vi "Save Material Theme.vi"(8 "error in":errorcluster, 10 "Theme":refnum<class "Material Theme.lvclass">, 11 "file path":path) -> (0 "error out":errorcluster, 1 "text":string)   [LabVIEW 2021, in "TSC Material Theme.lvlib" / "Material Theme.lvclass"]
doc: "Save a material theme from to disk in a JSON file format.\n\n<b>Code Developed By:</b> +\nTechnology Service Corporation +\nwww.tsc.com/atcs\n\nDeveloper:\nDaniel Coons"
uses:
  Material Theme.lvclass
  Material Theme.lvclass/Material Theme.ctl
  <vilib>/JDP Science/JSONtext/LVClass Serializer/JSONtext LVClass Serializer.lvclass
  TSC Material Theme.lvlib
  Material-Scheme/Material-Scheme.lvclass
  Material-Palette/Material-Palette.lvclass
  <vilib>/JDP Science/JSONtext/JSONtext.lvlib
  6cf305a8-b973-47b4-be4a-a40db0a30ff0.vi
panel:
  # "FOR DEBUG"
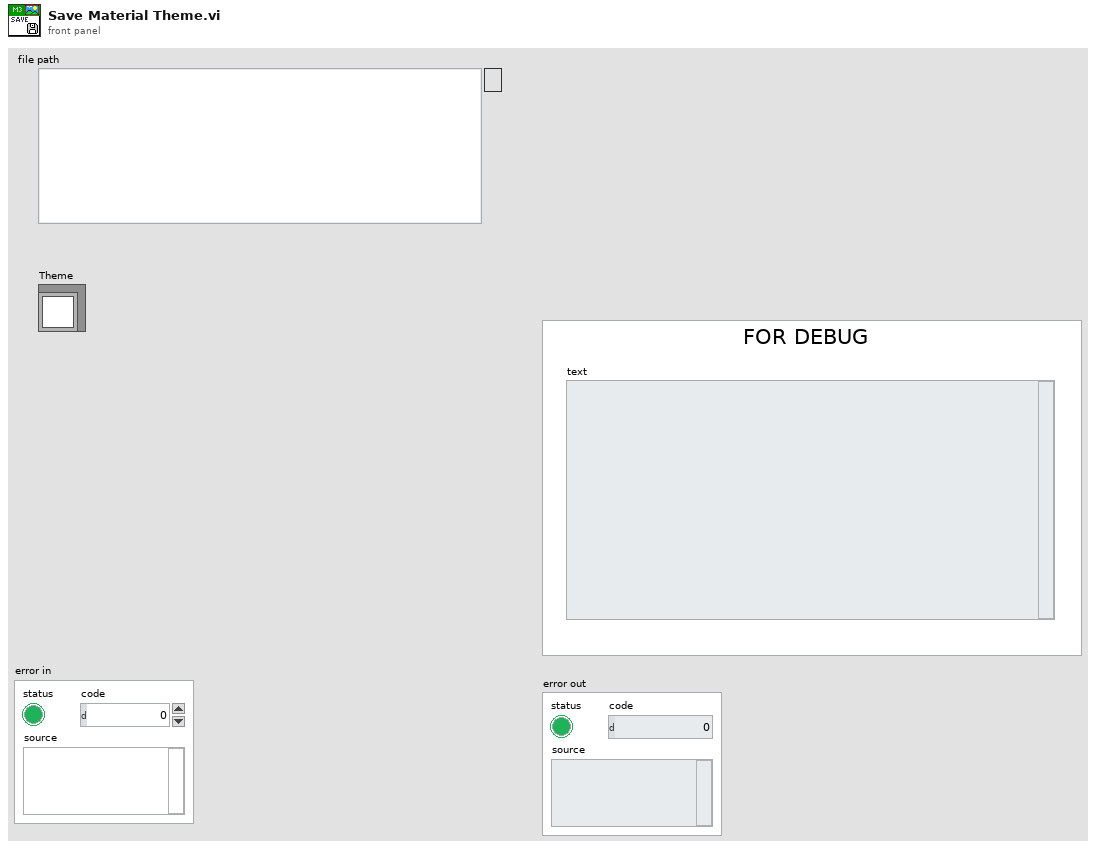
[diagram p1: front panel]
types:
  T1 = enum16{"open", "replace", "create", "open or create", "replace or create", "replace or create with confirmation"}
  T2 = cluster{"primary":u32, "secondary":u32, "tertiary":u32, "error":u32}
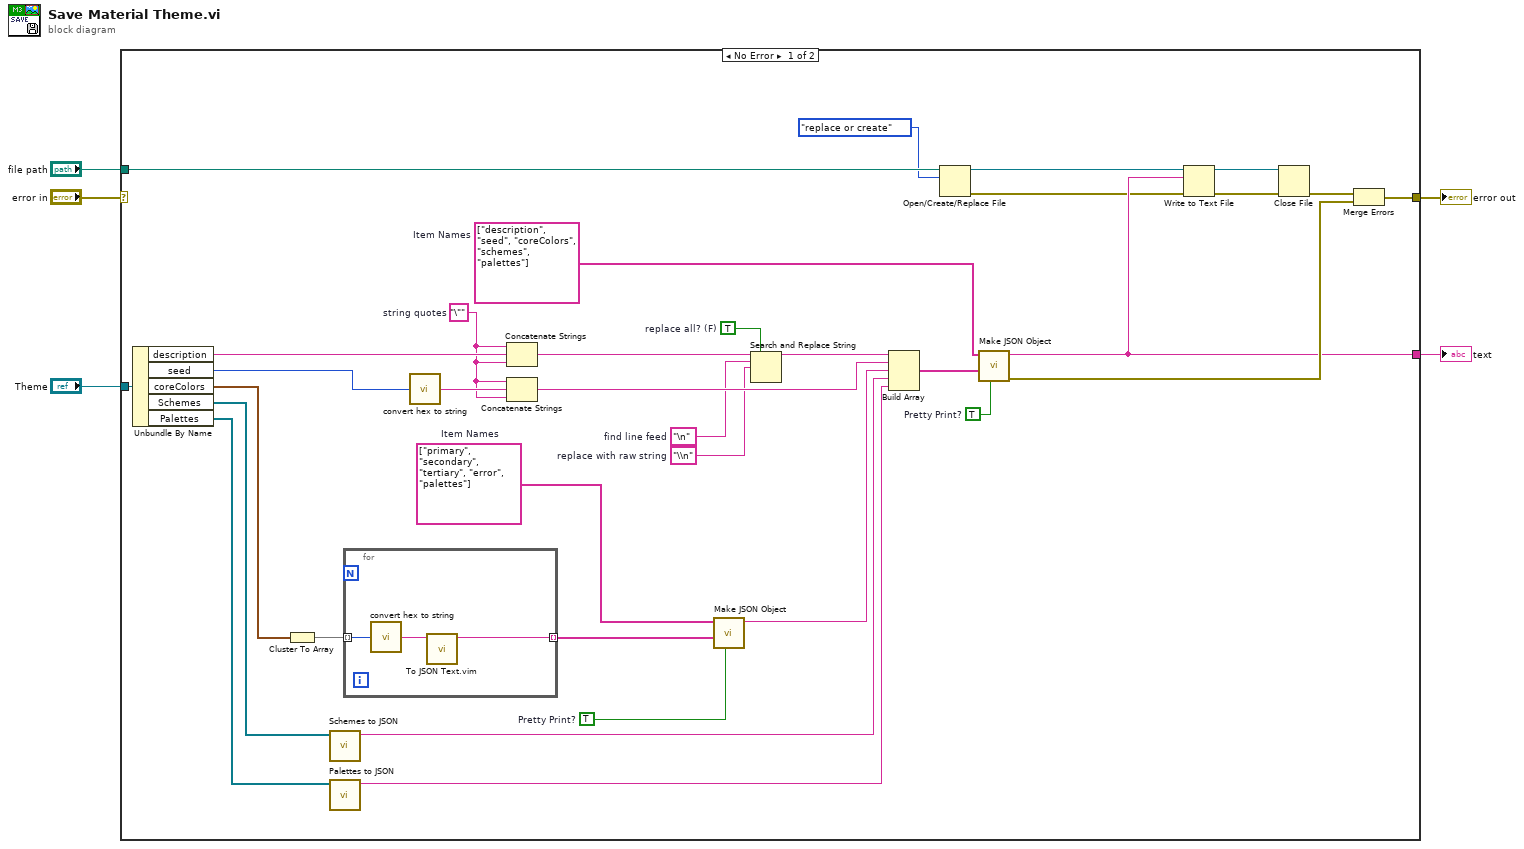
[diagram p0: block diagram]
diagram:
  n1 = case shown="No Error" "error in" {
    selector: "error in" -> [_ w43]
    tunnel: [w38 w43] -> w5
    tunnel: "file path" -> [w35 _]
    tunnel: "Theme" -> [w17 _]
    tunnel: [w15 _] -> w2
    frame No Error {
      w11 = "\\n"  # replace with raw string
      w12 = "\n"  # find line feed
      w13 = TRUE  # replace all? (F)
      w16 = TRUE  # Pretty Print?
      w19 = string[] ["primary", "secondary", "tertiary", "error", "palettes"]  # Item Names
      w24 = "\""  # string quotes
      w32 = string[] ["description", "seed", "coreColors", "schemes", "palettes"]  # Item Names
      w31 = TRUE  # Pretty Print?
      n2 = Unbundle By Name(w17) -> ("description"=w25:string, "seed"=w36:u32, "coreColors"=w20:T2, "Schemes"=w34:refnum<class "Material-Scheme.lvclass">[], "Palettes"=w33:refnum<class "Material-Palette.lvclass">[])
      n3 = Cluster To Array(cluster=w20) -> (array=w22:u32[])
      n4 = call "Schemes to JSON.vi"("Schemes"=w34) -> ("Material JSON"=w29:string)  [unwired: 9 in, 1 out]
      n5 = call "Palettes to JSON.vi"("Palettes"=w33) -> ("Material JSON"=w28:string)  [unwired: 9 in, 1 out]
      n6 = for {
        tunnel: [w42] -> w21 mode=indexing
        tunnel: w22 -> [w41] mode=indexing
        n7 = call "convert hex to string.vi"("hex"=w41) -> ("string"=w40:string)
        n8 = call "To JSON Text.vim"("Anything"=w40) -> ("<JSON>"=w42:string)  [unwired: 9 in, 1 out]
      }
      n9 = call "convert hex to string.vi"("hex"=w36) -> ("string"=w30:string)
      n10 = Concatenate Strings(w24, w25, w24) -> (w23:string)
      n11 = Concatenate Strings(w24, w30, w24) -> (w26:string)
      n12 = call <vilib>:"Make JSON Object.vi"("Pretty Print?"=w16, "JSON Items"=w21, "Item Names"=w19) -> ("<JSON>"=w18:string)  [unwired: 7 in, 1 out]
      n13 = Search and Replace String(replace all?=w13, input string=w23, search string=w12, replace string=w11) -> (result string=w14:string)  [unwired: 4 in, 3 out]
      n14 = Build Array(w14, w26, w18, w29, w28) -> (w27:string[])
      n15 = Open/Create/Replace File(file path (use dialog)=w35, operation (0:open)=T1."replace or create") -> (refnum out=w8:refnum<file>, error out=w10:errorcluster)  [unwired: 4 in, 1 out]
      n16 = call <vilib>:"Make JSON Object.vi"("Pretty Print?"=w31, "JSON Items"=w27, "Item Names"=w32) -> ("error out"=w37:errorcluster, "<JSON>"=w15:string)  [unwired: 7 in]
      n17 = Write to Text File(file (use dialog)=w8, text=w15, error in=w10) -> (refnum out=w7:refnum<file>, error out=w9:errorcluster)  [unwired: 1 in, 1 out]
      n18 = Close File(refnum=w7, error in=w9) -> (error out=w39:errorcluster)  [unwired: 1 out]
      n19 = Merge Errors(w39, w37) -> (w38:errorcluster)
    }
    frame Error {
      # "don't save if error"
    }
  }
  "error out" <- w5
  "text" <- w2
